vi "SVT Build Result Table.vi"   [LabVIEW 2017, in "SoundVib_Octave.lvlib"]
doc: "Generates a table of the results of a fractional-octave analysis. The first column of the table contains the nominal frequencies in Hz. The second and subsequent columns contain the 1/n band power with the appropriate unit label. Wire data to the <B>octave spectrum</B> input to determine the polymorphic instance to use or manually select the instance."
uses:
  <vilib>/addons/Sound and Vibration/svt_Octave/SoundVib_Octave.lvlib
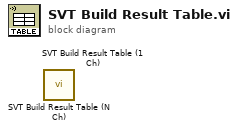
[diagram p0: block diagram]
diagram:
  n1 = call <vilib>:"SVT Build Result Table (N Ch).vi"() -> ()  [unwired: 13 in, 3 out]
  n2 = call <vilib>:"SVT Build Result Table (1 Ch).vi"() -> ()  [unwired: 13 in, 3 out]
